vi "Init Motor.vi"(7 "ENC Offset":dbl, 8 "error in (no error)":errorcluster caption="error in", 10 "Motor ID":u8, 11 "Port Selection Info In":T1={"Port Name"="", "Amplifier Num"=1, "Baud Rate"=38400, "Char Formation"=enum."0"} {"Baud Rate" items=["38400"=38400, "19200"=19200, "9600"=9600, "115200"=0]; "Amplifier Num" max=31}) -> (0 "error out":errorcluster, 3 "FujiMotor out":refnum<class "FujiMotor.lvclass">)   [LabVIEW 2014, in "ALPHA5 RS485.lvlib" / "FujiMotor.lvclass"]
uses:
  FujiMotor.lvclass
  typedefs/Port Selection Info.ctl
  FujiMotor.lvclass/FujiMotor.ctl
  ALPHA5 RS485.lvlib
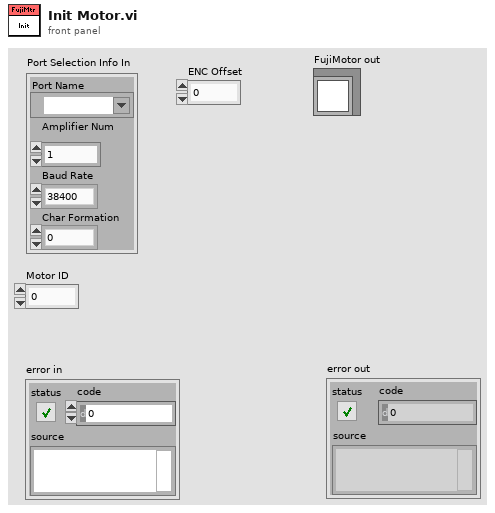
[diagram p1: front panel]
types:
  T1 = typedef "ALPHA5 RS485.lvlib/Port Selection Info.ctl" = cluster{"Port Name":refnum<visa-resource-name>, "Amplifier Num":u8, "Baud Rate":u32, "Char Formation":enum16{"0", "1", "2", "3", "4", "5"}}
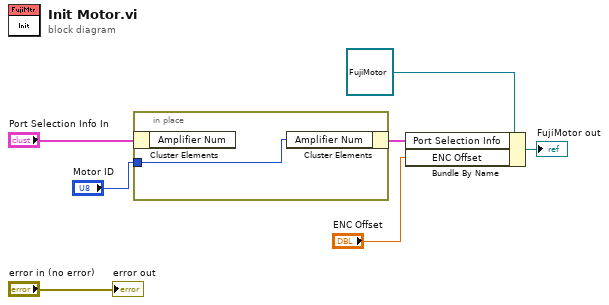
[diagram p0: block diagram]
diagram:
  n1 = in-place {
    in-place-border: "Motor ID" -> [w8]
    n2 = in-place-cluster #1("Port Selection Info In") -> ()  [unwired: 1 out]
    n3 = in-place-cluster #1("Amplifier Num"=w8) -> (w4:T1)
  }
  n4 = Bundle By Name(cluster=refnum<class "FujiMotor.lvclass"> refnum ("ALPHA5 RS485.lvlib:FujiMotor.lvclass"), "Port Selection Info"=w4, "ENC Offset"="ENC Offset") -> (→"FujiMotor out":refnum<class "FujiMotor.lvclass">)
  "error out" <- "error in (no error)"
